vi "Approx Equal.vi"(9 "Tolerance":dbl, 10 "b":dbl, 11 "a":dbl) -> (3 "a == b?":bool)   [LabVIEW 2018]
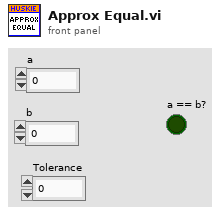
[diagram p1: front panel]
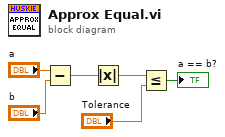
[diagram p0: block diagram]
diagram:
  n1 = Subtract(x="a", y="b") -> (x-y=w4:dbl)
  n2 = Absolute Value(x=w4) -> (abs(x)=w3:dbl)
  n3 = Less Or Equal?(x=w3, y="Tolerance") -> (x <= y?=→"a == b?":bool)
